vi "FPGA_PID.vi"() -> ()   [LabVIEW 2019]
uses:
  <vilib>/rvi/Analysis/control/PID/Typedef/niFpgaPID_ManualControl.ctl
  <vilib>/rvi/Analysis/control/PID/Typedef/niFpgaPID_OutputRange.ctl
  <vilib>/rvi/Analysis/control/PID/Typedef/niFpgaPID_PIDGains.ctl
  <vilib>/rvi/Emulation/niFpgaGetClockAttributes.vi
  <vilib>/rvi/Emulation/niFpgaSctlEmulationGetInTimedLoop.vi
  <vilib>/rvi/Emulation/niFpgaEmulationReportErrorSimple.vi
  <vilib>/rvi/Analysis/control/PID/SubVIs/niFpgaPID_PIDWrapper.vi
  <vilib>/rvi/Emulation/niFpgaCriticalErrorInLSC.vi
panel:
  in  "stop":bool
  out "output":sgl
  in  "gains":T1 {"filter coefficient" min=0 max=1; "proportional gain" step=0.125}
  in  "output range":T2={"output high (Inf)"=inf, "output low (-Inf)"=-inf}
  in  "manual control":T3
  in  "process variable":sgl
  in  "setpoint":sgl
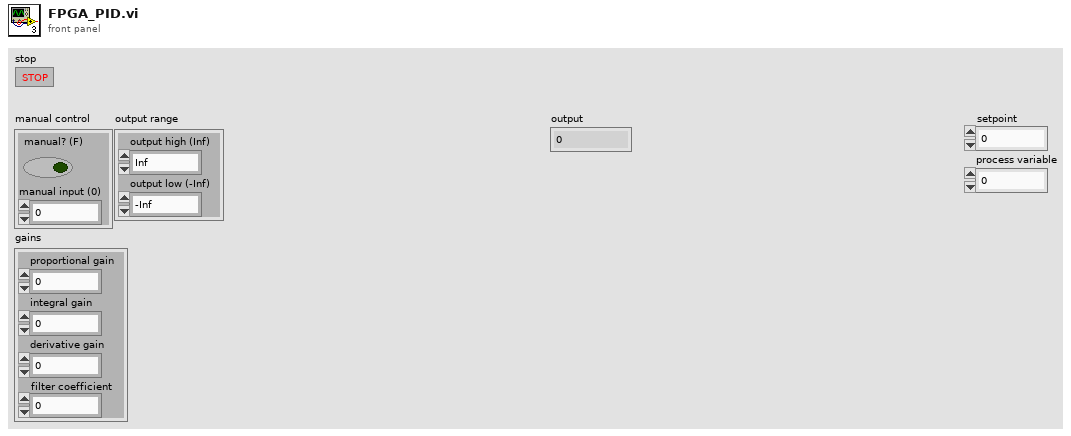
[diagram p1: front panel]
types:
  T1 = typedef "niFpgaPID_PIDGains.ctl" = cluster{"proportional gain":sgl, "integral gain":sgl, "derivative gain":sgl, "filter coefficient":sgl}
  T2 = typedef "niFpgaPID_OutputRange.ctl" = cluster{"output high (Inf)":sgl, "output low (-Inf)":sgl}
  T3 = typedef "niFpgaPID_ManualControl.ctl" = cluster{"manual? (F)":bool, "manual input (0)":sgl}
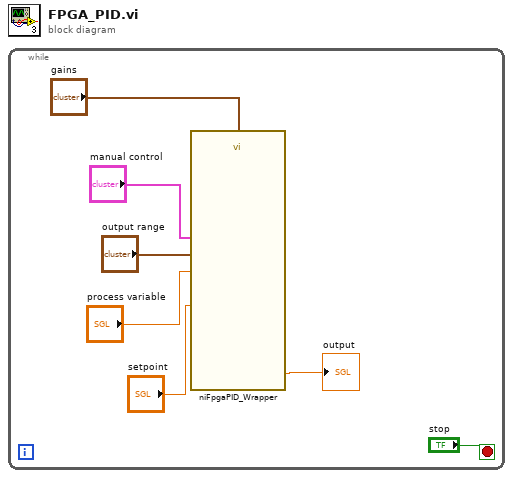
[diagram p0: block diagram]
diagram:
  n1 = while {
    stop <- "stop" stop-if-true
    n2 = call-poly <vilib>:"niFpgaPID_Wrapper.vi"("setpoint"="setpoint", "process variable"="process variable", "manual control"="manual control", "gains"="gains", "output range"="output range") -> ("output"=→"output":sgl)  [unwired: 8 in, 2 out]
  }
